vi "ImagePositionToSample (SubVI).vi"(4 "image_y":u16, 5 "image size_y":u16, 6 "image_x":u16, 7 "image size_x":u16, 8 "sample end_y":fxp<+/-,26,5>, 9 "sample end_x":fxp<+/-,26,5>, 10 "sample start_y":fxp<+/-,26,5>, 11 "sample start_x":fxp<+/-,26,5>) -> (0 "sample_y":fxp<+/-,26,5>, 1 "sample_x":fxp<+/-,26,5>, 2 "increment_y":fxp<+/-,26,5>, 3 "increment_x":fxp<+/-,26,5>)   [LabVIEW 2017]
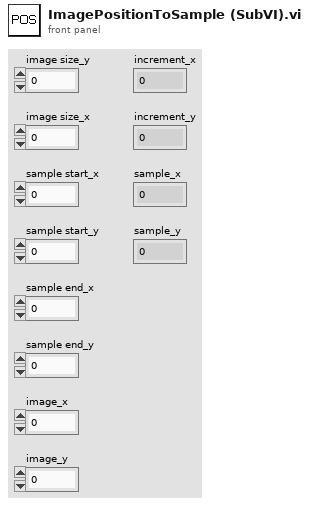
[diagram p1: front panel]
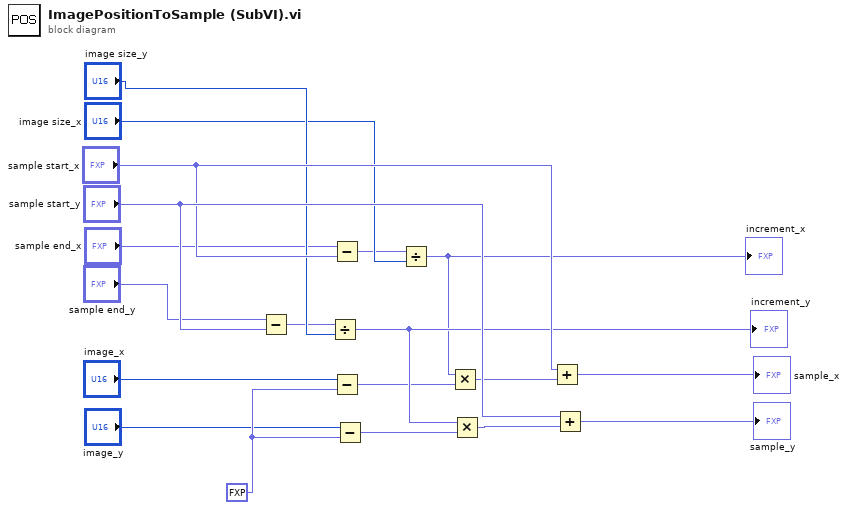
[diagram p0: block diagram]
diagram:
  w9 = fxp<+,1,0> 0.5 ("y")
  n1 = Subtract(x="sample end_y", y="sample start_y") -> (x-y=w4:fxp<+/-,27,6>)
  n2 = Divide(x=w4, y="image size_y") -> (x/y=w13:fxp<+/-,43,6>)
  "increment_y" <- w13
  n3 = Subtract(x="sample end_x", y="sample start_x") -> (x-y=w2:fxp<+/-,27,6>)
  n4 = Subtract(x="image_x", y=w9) -> (x-y=w11:fxp<+/-,18,17>)
  n5 = Subtract(x="image_y", y=w9) -> (x-y=w12:fxp<+/-,18,17>)
  n6 = Divide(x=w2, y="image size_x") -> (x/y=w10:fxp<+/-,43,6>)
  "increment_x" <- w10
  n7 = Multiply(x=w10, y=w11) -> (x*y=w14:fxp<+/-,60,22>)
  n8 = Multiply(x=w13, y=w12) -> (x*y=w16:fxp<+/-,60,22>)
  n9 = Add(x="sample start_x", y=w14) -> (x+y=→"sample_x":fxp<+/-,60,22>)
  n10 = Add(x="sample start_y", y=w16) -> (x+y=→"sample_y":fxp<+/-,60,22>)
